vi "NI 9215.vi"(2 "sample mode":i32(ring)=10178 items=["Finite Samples"=10178, "Continuous Samples"=10123, "Hardware Timed Single Point"=12522], 3 "MODULE 3 (0-10V)":string="CDR_AI", 4 "rate":dbl=1000.0 format="%0.2f", 5 "error in":errorcluster) -> (14 "task out":refnum<k21>, 19 "error out":errorcluster)   [LabVIEW 2019]
uses:
  <vilib>/DAQmx/configure/timing.llb/DAQmx Timing (Sample Clock).vi
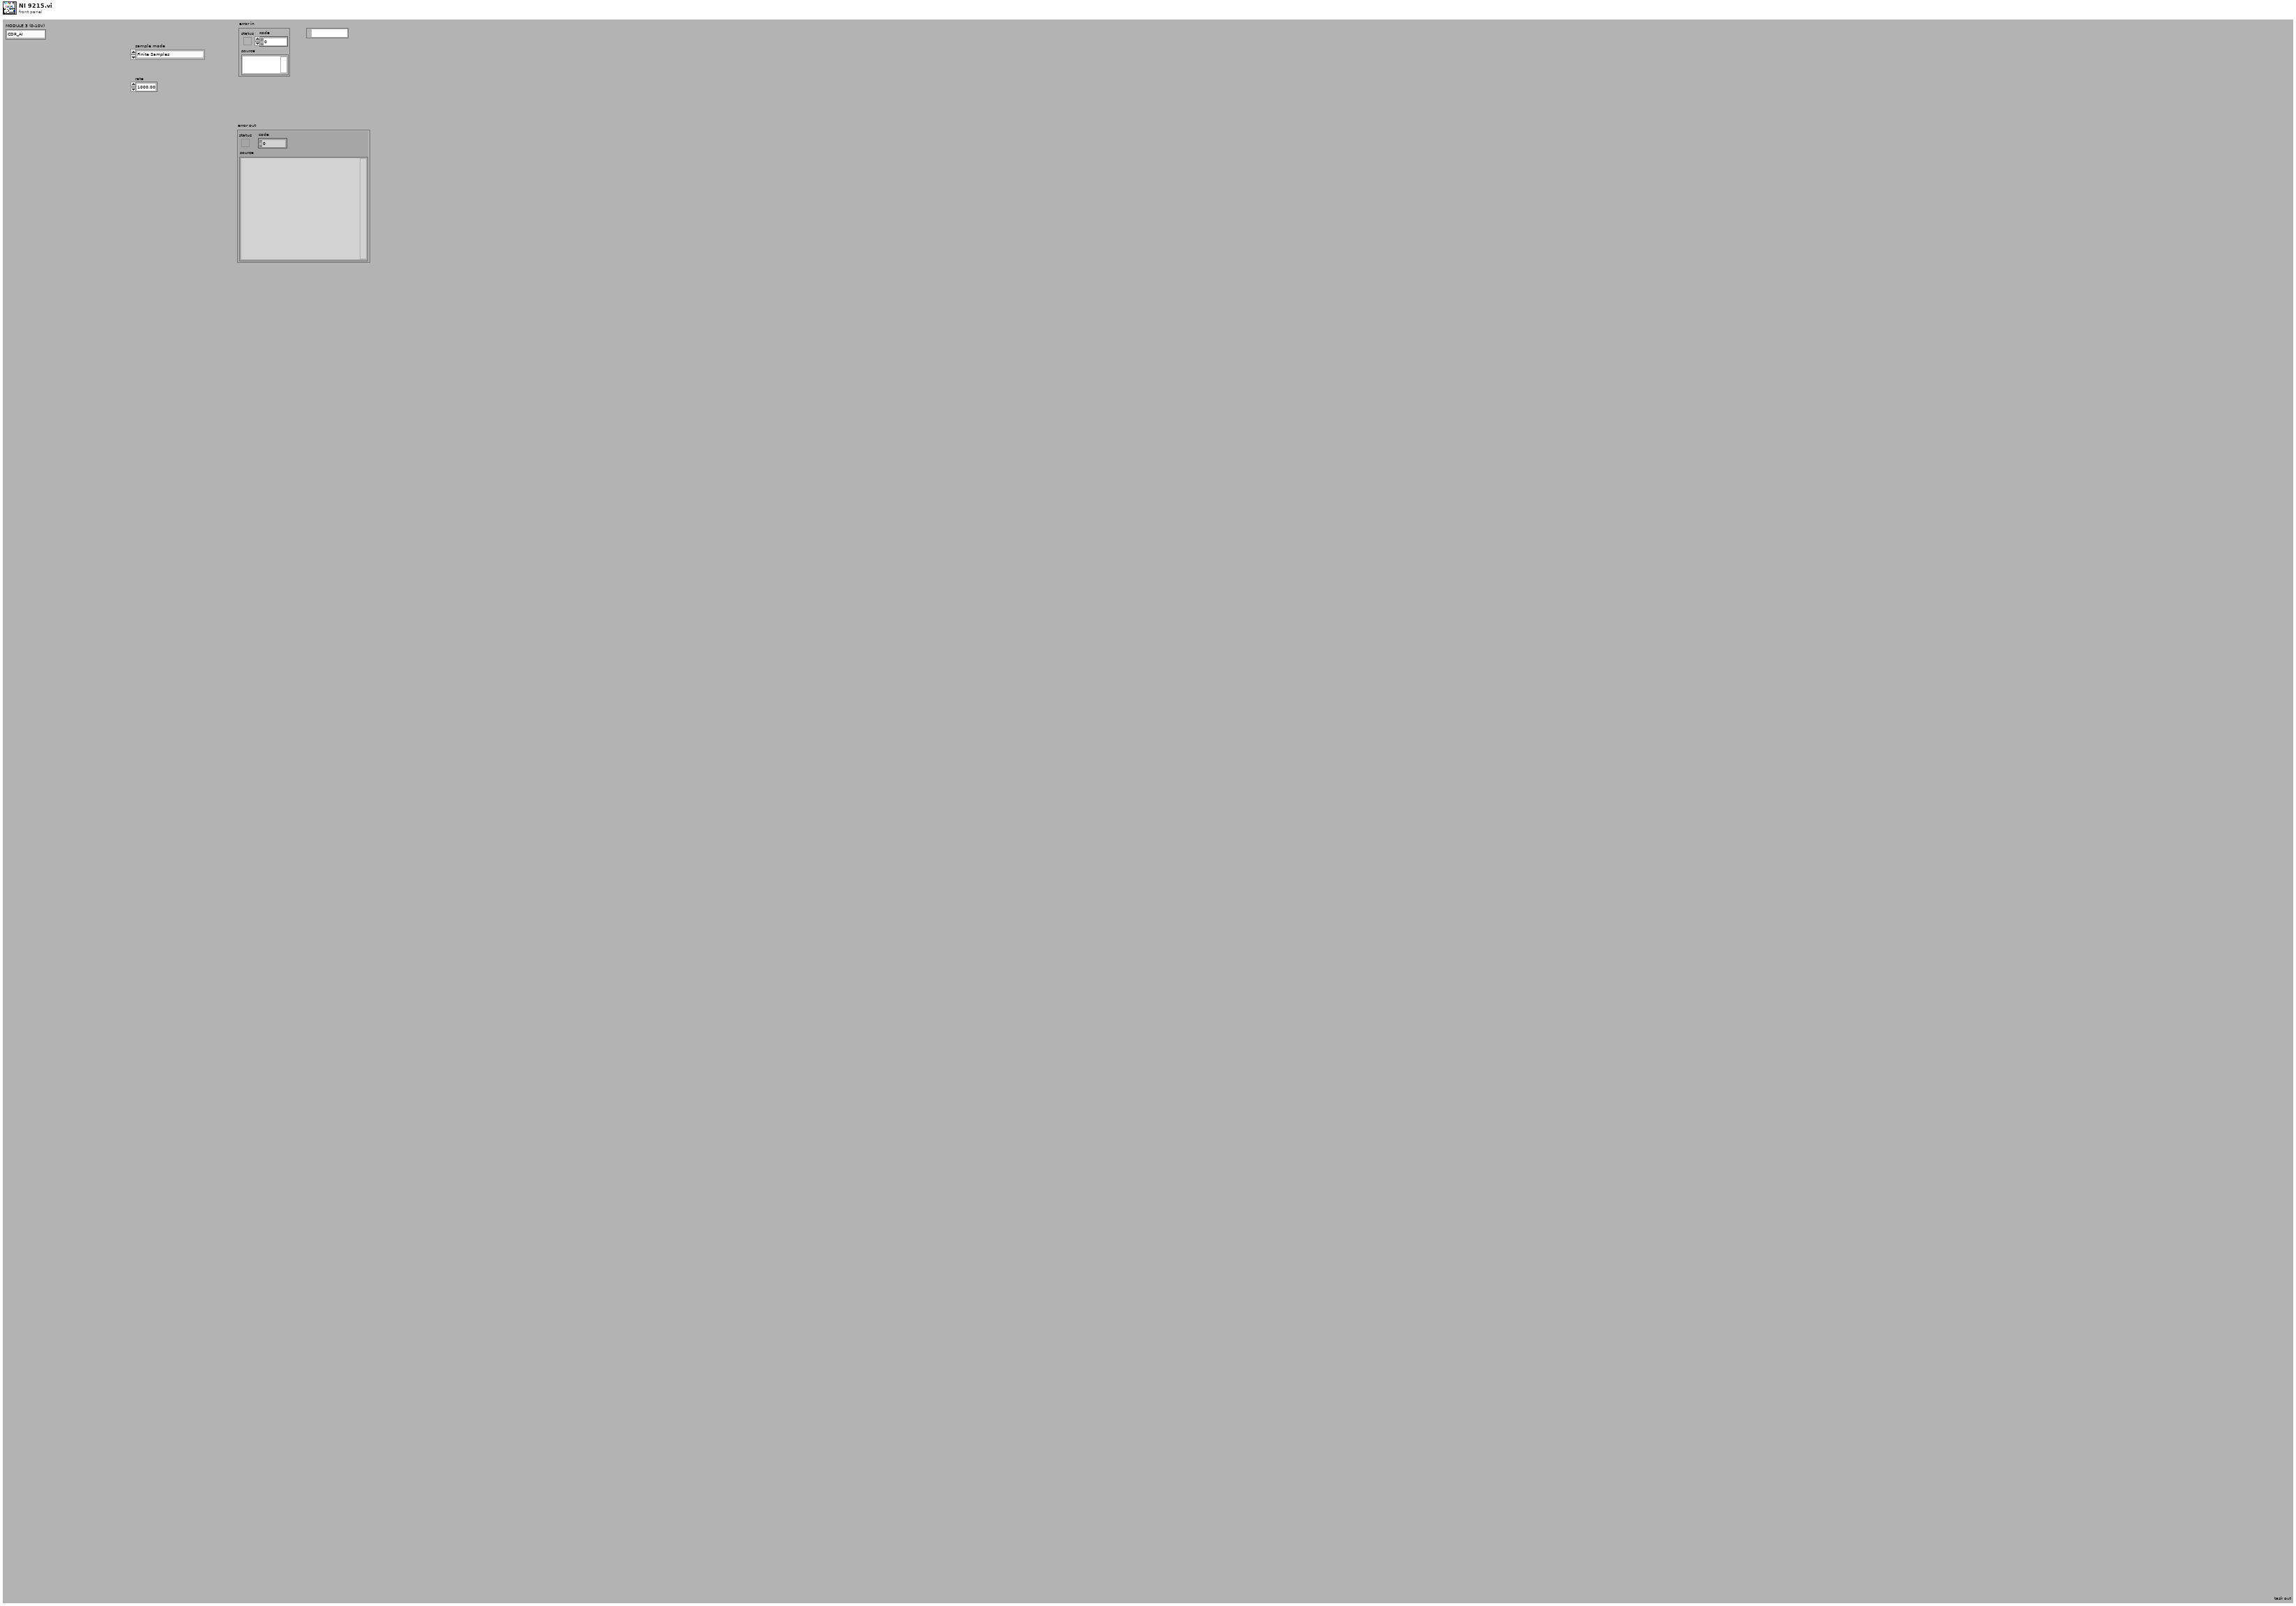
[diagram p1: front panel]
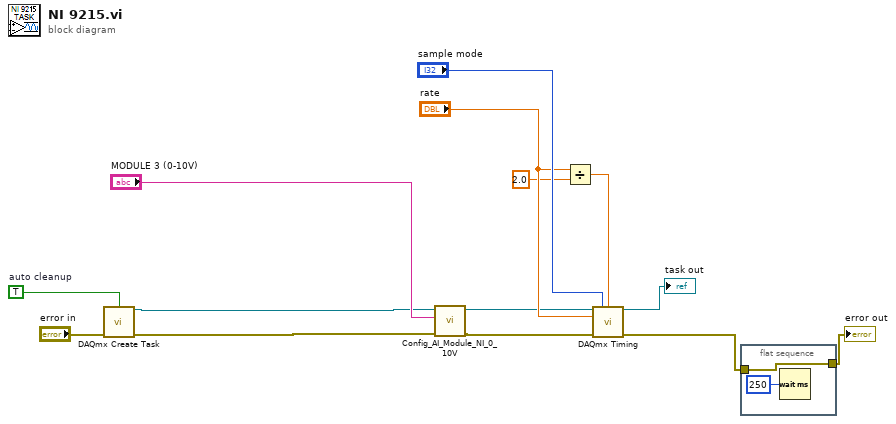
[diagram p0: block diagram]
diagram:
  w13 = TRUE  # auto cleanup
  n1 = call <vilib>:"DAQmx Create Task.vi"("auto cleanup"=w13, "error in"="error in") -> ("task out"=w2:refnum<k21>, "error out"=w1:errorcluster)  [unwired: 12 in]
  n2 = call "Config_AI_Module_NI_0_10V.vi"("error in (no error)"=w1, "MODULE NAME"="MODULE 3 (0-10V)", "Refnum in"=w2) -> ("error out"=w4:errorcluster, "Refnum out"=w3:refnum<k21>)  [unwired: 7 in]
  n3 = Divide(x="rate", y=2.0) -> (x/y=w8:dbl)
  n4 = call-poly <vilib>:"DAQmx Timing.vi"("task/channels in"=w3, "sample mode"="sample mode", "samples per channel"=w8, "rate"="rate", "error in"=w4) -> ("task out"=→"task out":refnum<k21>, "error out"=w7:errorcluster)  [unwired: 9 in]
  n5 = flat-sequence {
    tunnel: [w15] -> w6
    tunnel: w7 -> [w15]
    frame #0 {
      n6 = Wait (ms)(milliseconds to wait=u32 250) -> ()  [unwired: 1 out]
    }
  }
  "error out" <- w6
